vi "RampSetting.vi"(1 "set/get":bool, 2 "RampSetting (in)":T1={"used"=FALSE, "steps"=2, "start (V)"=0.0, "stop (V)"=0.0, "periode (s)"=30.0, "manual"=[]} {"periode (s)" min=0.001; "stop (V)" min=0.0 max=10.0; "start (V)" min=0.0 max=10.0; "steps" min=1 step=1}) -> (0 "RampSetting (out)":T1={"used"=FALSE, "steps"=2, "start (V)"=0.0, "stop (V)"=0.0, "periode (s)"=30.0, "manual"=[]} {"periode (s)" min=0.001; "stop (V)" min=0.0 max=10.0; "start (V)" min=0.0 max=10.0; "steps" min=1 step=1})   [LabVIEW 2009]
doc: "Dieses VI dient als Variable mit den Einstellungen für die Betriebsart \"Intensitäts-Rampe\"."
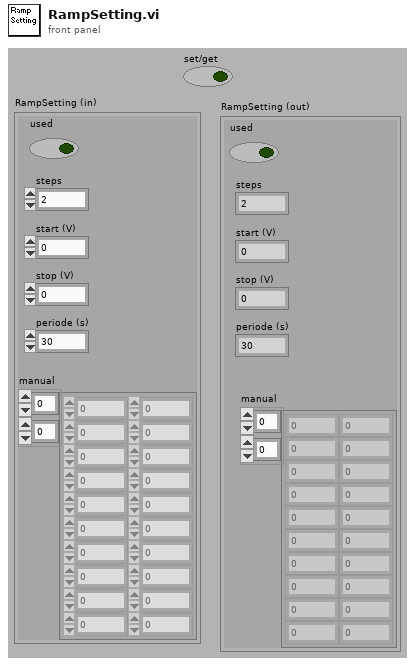
[diagram p1: front panel]
types:
  T1 = cluster{"used":bool, "steps":u16, "start (V)":dbl, "stop (V)":dbl, "periode (s)":dbl, "manual":dbl[][]}
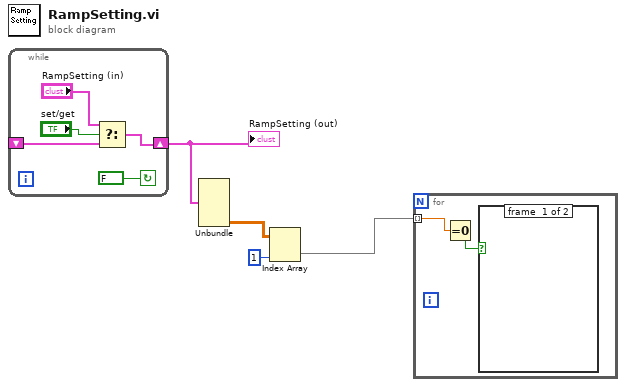
[diagram p0: block diagram]
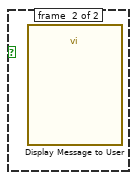
[diagram p2: hidden frame]
diagram:
  n1 = while {
    shift-right: [w6] -> w4
    shift-left: _ -> [w5]
    stop <- FALSE continue-if-true
    n2 = Select(t="RampSetting (in)", s="set/get", f=w5) -> (s? t:f=w6:T1)
  }
  "RampSetting (out)" <- w4
  n3 = Unbundle(w4) -> ("manual"=w3:dbl[][])  [unwired: 5 out]
  n4 = Index Array(array=w3, index (col)=1 ("disabled index (col)")) -> (element=w1:dbl[])  [unwired: 1 in]
  n5 = for {
    tunnel: w1 -> [w11] mode=indexing
    n6 = Equal To 0?(x=w11) -> (x = 0?=w10:bool)
    n7 = case shown="True" w10 {
      frame #0 {
      }
      frame #1 {
        n8 = call "Display Message to User"() -> ()  [unwired: 10 in, 2 out]
      }
    }
  }
